vi "CreateLogFiles.vi"(8 "error in (no error)":errorcluster) -> (0 "error out":errorcluster, 1 "Tdms log file":refnum<k34>, 3 "Txt log file":refnum<file>)   [LabVIEW 2020]
doc: "Creates txt file with Maestro communcation logs and tdms file with servo positions logs based on directories from config file. If there is no config file or paths are not specified, logs are created in application directory."
uses:
  <vilib>/Utility/config.llb/Read Key (Path).vi
  <vilib>/Utility/config.llb/NI_LVConfig.lvlib
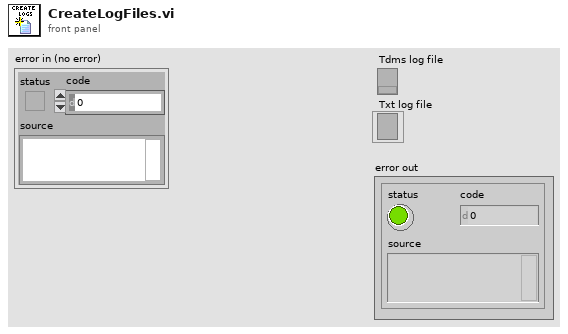
[diagram p1: front panel]
types:
  T1 = enum16{"open", "open or create", "create or replace", "create", "open (read-only)"}
  T2 = enum16{"open", "replace", "create", "open or create", "replace or create", "replace or create with confirmation"}
  T3 = typedef "NI_LVConfig.lvlib/Config Data RefNum.ctl" = refnum<k1>
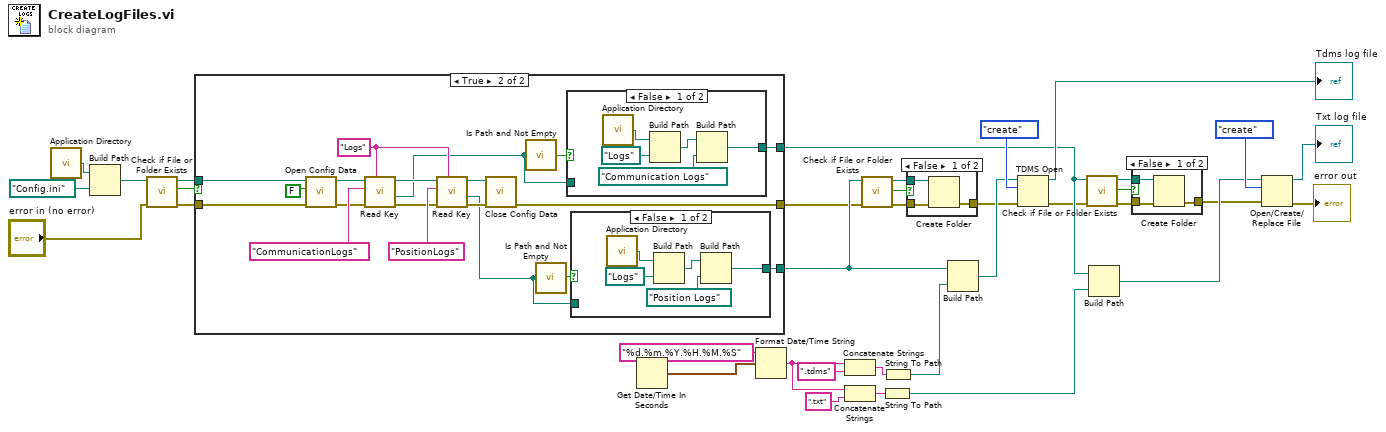
[diagram p0: block diagram]
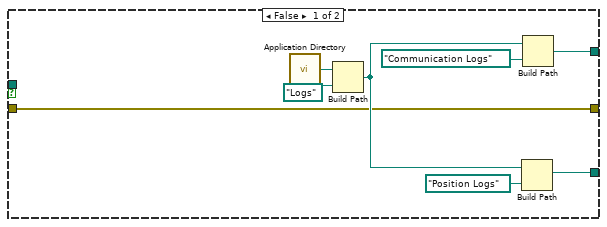
[diagram p2: hidden frame]
diagram:
  n1 = call <vilib>:"Application Directory.vi"() -> ("Application Directory"=w29:path)
  n2 = Build Path(base path=w29, name or relative path=path "Config.ini") -> (appended path=w7:path)
  n3 = call <vilib>:"Check if File or Folder Exists.vi"("error in (no error)"="error in (no error)", "path"=w7) -> ("error out"=w3:errorcluster, "file or folder exists?"=w6:bool, "dup path"=w5:path)  [unwired: 7 in]
  n4 = case shown="True" w6 {
    tunnel: [w40 w49] -> w17
    tunnel: [w41 w48] -> w9
    tunnel: w5 -> [_ w46]
    tunnel: w3 -> [w36 w45]
    tunnel: [w36 w47] -> w2
    frame False {
      n5 = call <vilib>:"Application Directory.vi"() -> ("Application Directory"=w39:path)
      n6 = Build Path(base path=w39, name or relative path=path "Logs") -> (appended path=w38:path)
      n7 = Build Path(base path=w38, name or relative path=path "Position Logs") -> (appended path=w40:path)
      n8 = Build Path(base path=w38, name or relative path=path "Communication Logs") -> (appended path=w41:path)
    }
    frame True {
      w59 = "Logs" ("section")
      n9 = call <vilib>:"Open Config Data.vi"("error in (no error)"=w45, "create file if necessary (T)"=FALSE, "configuration file path"=w46) -> ("error out"=w55:errorcluster, "refnum"=w54:T3)  [unwired: 6 in, 1 out]
      n10 = call-poly <vilib>:"Read Key.vi"("section"=w59, "error in (no error)"=w55, "key"="CommunicationLogs", "refnum"=w54) -> ("error out"=w57:errorcluster, "value"=w50:path, "refnum out"=w58:T3)  [unwired: 4 in, 1 out]
      n11 = call-poly <vilib>:"Read Key.vi"("section"=w59, "error in (no error)"=w57, "key"="PositionLogs", "refnum"=w58) -> ("error out"=w62:errorcluster, "value"=w44:path, "refnum out"=w61:T3)  [unwired: 4 in, 1 out]
      n12 = call <vilib>:"Close Config Data.vi"("error in (no error)"=w62, "refnum"=w61) -> ("error out"=w47:errorcluster)  [unwired: 8 in, 1 out]
      n13 = call <vilib>:"Is Path and Not Empty.vi"("path"=w50) -> ("Is Path and Not Empty?"=w51:bool)  [unwired: 4 in]
      n14 = call <vilib>:"Is Path and Not Empty.vi"("path"=w44) -> ("Is Path and Not Empty?"=w52:bool)  [unwired: 4 in]
      n15 = case shown="False" w51 {
        tunnel: [w63 w68] -> w48
        tunnel: w50 -> [_ w68]
        frame False {
          n16 = call <vilib>:"Application Directory.vi"() -> ("Application Directory"=w64:path)
          n17 = Build Path(base path=w64, name or relative path=path "Logs") -> (appended path=w65:path)
          n18 = Build Path(base path=w65, name or relative path=path "Communication Logs") -> (appended path=w63:path)
        }
        frame True {
        }
      }
      n19 = case shown="False" w52 {
        tunnel: [w69 w74] -> w49
        tunnel: w44 -> [_ w74]
        frame False {
          n20 = call <vilib>:"Application Directory.vi"() -> ("Application Directory"=w70:path)
          n21 = Build Path(base path=w70, name or relative path=path "Logs") -> (appended path=w71:path)
          n22 = Build Path(base path=w71, name or relative path=path "Position Logs") -> (appended path=w69:path)
        }
        frame True {
        }
      }
    }
  }
  n23 = Get Date/Time In Seconds() -> (seconds since 1Jan1904=w26:timestamp)
  n24 = Format Date/Time String(time format string (%c)="%d.%m.%Y.%H.%M.%S", seconds (now)=w26) -> (date/time string=w21:string)  [unwired: 1 in]
  n25 = Concatenate Strings(w21, ".tdms" ("string")) -> (w19:string)
  n26 = Concatenate Strings(w21, ".txt" ("string")) -> (w32:string)
  n27 = call <vilib>:"Check if File or Folder Exists.vi"("error in (no error)"=w2, "path"=w17) -> ("error out"=w16:errorcluster, "file or folder exists?"=w14:bool, "dup path"=w15:path)  [unwired: 7 in]
  n28 = String To Path(string=w32) -> (path=w31:path)
  n29 = String To Path(string=w19) -> (path=w18:path)
  n30 = case shown="False" w14 {
    tunnel: w16 -> [w77 w78]
    tunnel: w15 -> [w76 _]
    tunnel: [w75 w78] -> w13
    frame False {
      n31 = Create Folder(path (use dialog)=w76, error in=w77) -> (error out=w75:errorcluster)  [unwired: 1 in, 2 out]
    }
    frame True {
    }
  }
  n32 = Build Path(base path=w17, name or relative path=w18) -> (appended path=w22:path)
  n33 = TDMS Open(8:w13, 10:T1."create" ("operation (0:open)"), 11:w22) -> (0:w1:errorcluster, 3:→"Tdms log file":refnum<k34>)  [unwired: 4 in]
  n34 = call <vilib>:"Check if File or Folder Exists.vi"("error in (no error)"=w1, "path"=w9) -> ("error out"=w12:errorcluster, "file or folder exists?"=w10:bool, "dup path"=w11:path)  [unwired: 7 in]
  n35 = Build Path(base path=w9, name or relative path=w31) -> (appended path=w28:path)
  n36 = case shown="False" w10 {
    tunnel: w12 -> [w81 w82]
    tunnel: w11 -> [w80 _]
    tunnel: [w79 w82] -> w8
    frame False {
      n37 = Create Folder(path (use dialog)=w80, error in=w81) -> (error out=w79:errorcluster)  [unwired: 1 in, 2 out]
    }
    frame True {
    }
  }
  n38 = Open/Create/Replace File(file path (use dialog)=w28, error in=w8, operation (0:open)=T2."create") -> (refnum out=→"Txt log file":refnum<file>, error out=→"error out":errorcluster)  [unwired: 3 in, 1 out]
